vi "SPI Coerce Frequency.vi"(10 "Frequency":dbl, 11 "Frequency Unit":enum16{"Hz", "KHz", "MHz"}(ring)) -> (2 "Actual Frequency (Hz)":dbl, 3 "Coerced Frequency?":bool)   [LabVIEW 2021]
uses:
  <vilib>/myRIO/Common/Instrument Driver Framework/myRIO v1.0/SPI/typedefs/SPI Configuration v1.0.ctl
  <vilib>/myRIO/Common/Instrument Driver Framework/myRIO v1.0/SPI/typedefs/SPI Clock Phase.ctl
  <vilib>/myRIO/Common/Instrument Driver Framework/myRIO v1.0/SPI/typedefs/SPI Clock Polarity.ctl
  <vilib>/myRIO/Common/Instrument Driver Framework/myRIO v1.0/SPI/typedefs/SPI Data Direction.ctl
  <vilib>/myRIO/Common/Instrument Driver Framework/myRIO v1.0/SPI/typedefs/SPI Frame Length.ctl
  <vilib>/myRIO/Common/Instrument Driver Framework/Utilities/vis/Calculate Clock Settings.vi
  <vilib>/myRIO/Common/Instrument Driver Framework/Utilities/vis/Calculate TOP (Phase Correct Mode).vi
  <vilib>/myRIO/Common/Instrument Driver Framework/Utilities/vis/Calculate TOP (Normal Mode).vi
  <vilib>/myRIO/Common/Instrument Driver Framework/Utilities/vis/Calculate Frequency (Phase Correct Mode).vi
  <vilib>/myRIO/Common/Instrument Driver Framework/Utilities/vis/Calculate Frequency (Normal Mode).vi
  <vilib>/Utility/error.llb/Error Cluster From Error Code.vi
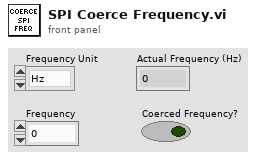
[diagram p1: front panel]
types:
  T1 = typedef "SPI Configuration v1.0.ctl" = cluster{"Frequency (Hz)":dbl, "SPI Clock Phase":T2, "SPI Clock Polarity":T3, "SPI Data Direction":T4, "Frame Length":T5}
  T2 = typedef "SPI Clock Phase.ctl" = enum8{"Leading", "Trailing"}
  T3 = typedef "SPI Clock Polarity.ctl" = enum8{"Low", "High"}
  T4 = typedef "SPI Data Direction.ctl" = enum8{"Most significant bit first", "Least significant bit first"}
  T5 = typedef "SPI Frame Length.ctl" = u8
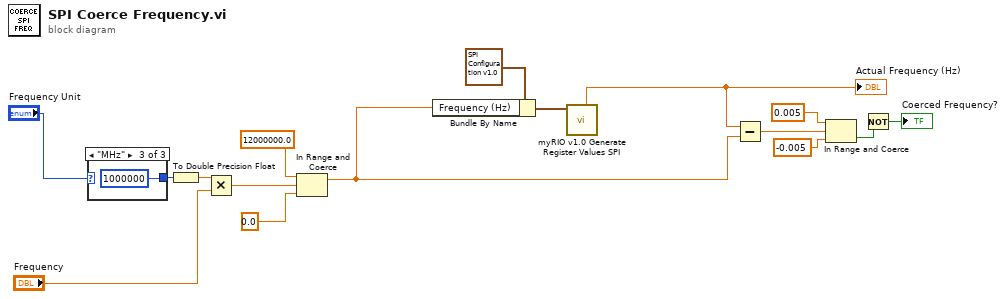
[diagram p0: block diagram]
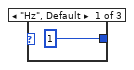
[diagram p2: hidden frame]
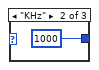
[diagram p3: hidden frame]
diagram:
  n1 = case shown="\"MHz\"" "Frequency Unit" {
    tunnel: [1 1000 1000000] -> w2
    frame "Hz", Default {
    }
    frame "KHz" {
    }
    frame "MHz" {
    }
  }
  n2 = To Double Precision Float(number=w2) -> (double precision float=w3:dbl)
  n3 = Multiply(x=w3, y="Frequency") -> (x*y=w4:dbl)
  n4 = In Range and Coerce(upper limit=12000000.0, x=w4, lower limit=0.0) -> (coerced(x)=w9:dbl)  [unwired: 1 out]
  n5 = Bundle By Name(cluster=T1 {"Frequency (Hz)"=0.0, "SPI Clock Phase"=enum."Leading", "SPI Clock Polarity"=enum."Low", "SPI Data Direction"=enum."Most significant bit first", "Frame Length"=1} ("SPI Configuration v1.0"), "Frequency (Hz)"=w9) -> (w13:T1)
  n6 = call <vilib>:"myRIO v1.0 Generate Register Values SPI.vi"("SPI Configuration v1.0"=w13) -> ("Actual Frequency (Hz)"=w15:dbl)  [unwired: 7 in, 3 out]
  "Actual Frequency (Hz)" <- w15
  n7 = Subtract(x=w15, y=w9) -> (x-y=w5:dbl)
  n8 = In Range and Coerce(upper limit=0.005, x=w5, lower limit=-0.005) -> (In Range?=w8:bool)  [unwired: 1 out]
  n9 = Not(x=w8) -> (.not. x?=→"Coerced Frequency?":bool)
